vi "PT 100 Temp Convert to R.vi"(6 "γ":dbl=4.2735e-12 format="%#_6e", 9 "β":dbl=-5.80195e-07 format="%#_6e", 10 "α":dbl=0.00390802 format="%#_6e", 11 "t":dbl) -> (3 "Rt":dbl)   [LabVIEW 2012]
doc: "功能：\n\n计算温度t大于等于0，且小于等于850时的RTD电阻值。"
uses:
  <vilib>/express/express arith-compare/Formula/XNode/ExpressFormulaBlockNode.xnode
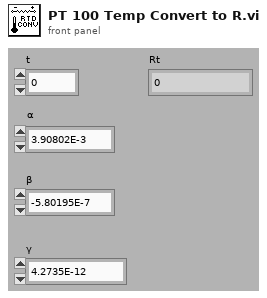
[diagram p1: front panel]
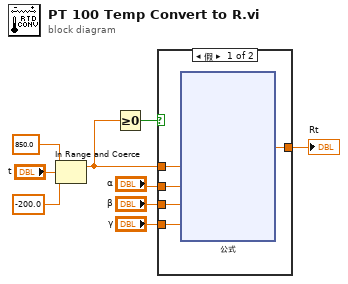
[diagram p0: block diagram]
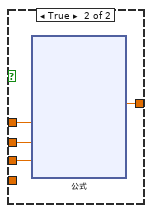
[diagram p2: hidden frame]
diagram:
  n1 = In Range and Coerce(upper limit=850.0 ("上限"), x="t", lower limit=-200.0 ("下限")) -> (coerced(x)=w4:dbl)  [unwired: 1 out]
  n2 = Greater Or Equal To 0?(x=w4) -> (x >= 0?=w6:bool)
  n3 = case shown="假" w6 {
    tunnel: [w14 w32] -> w5
    tunnel: w4 -> [w13 w31]
    tunnel: "α" -> [w12 w30]
    tunnel: "β" -> [w11 w29]
    tunnel: "γ" -> [w10 _]
    frame False {
      n4 = xnode "公式"("t"=w13, "A"=w12, "B"=w11, "C"=w10) -> ("结果"=w14:dbl)  [unwired: 1 in, 1 out]
    }
    frame True {
      n5 = xnode "公式"("t"=w31, "A"=w30, "B"=w29) -> ("结果"=w32:dbl)  [unwired: 1 in, 1 out]
    }
  }
  "Rt" <- w5
